vi "Master VI.vi"() -> ()   [LabVIEW 2014]
panel:
  in  "stop":bool
  in  "Knob":dbl(knob) scale=0.0..10.0
  in  "Button":bool
  # "SHARED VARIABLE"
  # "BUTTON"
  # "KNOB"
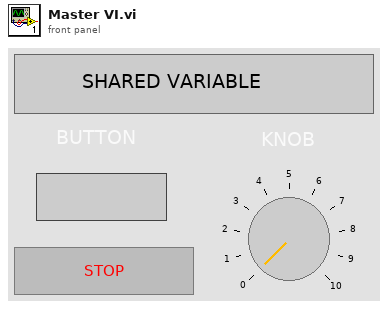
[diagram p1: front panel]
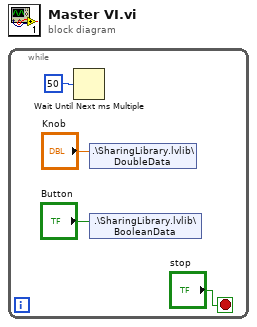
[diagram p0: block diagram]
diagram:
  n1 = while {
    stop <- "stop" stop-if-true
    n2 = Wait Until Next ms Multiple(millisecond multiple=u32 50) -> ()  [unwired: 1 out]
    n3 = shared-variable ".\\SharingLibrary.lvlib\\DoubleData"("Knob") -> ()  [unwired: 1 in, 1 out]
    n4 = shared-variable ".\\SharingLibrary.lvlib\\BooleanData"("Button") -> ()  [unwired: 1 in, 1 out]
  }
